vi "iLoveLangmuirProbes.vi"() -> ()   [LabVIEW 2022 SP3]
panel:
  out "Numeric":dbl
  out "Waveform Graph":dynamicdata(graph)
  out "XY Graph":cluster{"Y":dbl[], "Y":dbl[]}[](graph)
  out "VBias":dbl(knob) scale=-10.0..10.0
  in  "stop":bool
  out "VR":dbl(knob) scale=-10.0..10.0
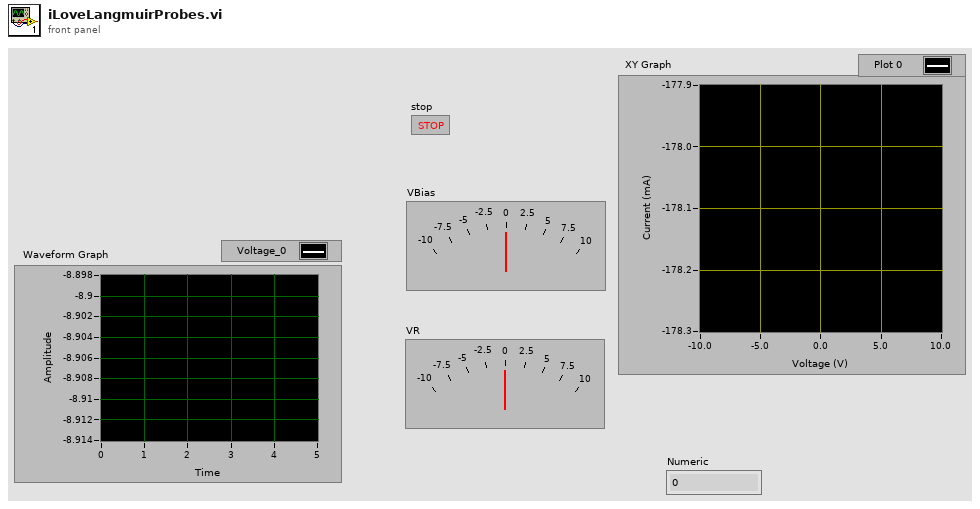
[diagram p1: front panel]
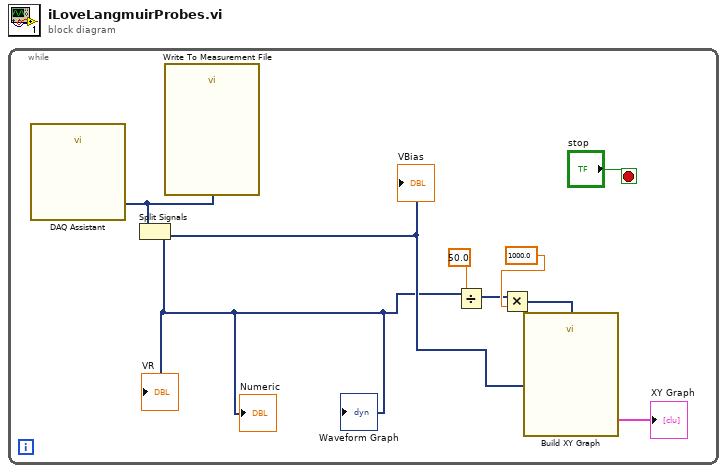
[diagram p0: block diagram]
diagram:
  n1 = while {
    stop <- "stop" stop-if-true
    n2 = call "DAQ Assistant"() -> ("data"=w3:dynamicdata)  [unwired: 17 in, 2 out]
    n3 = Split Signals(w3) -> (w1:dynamicdata, w2:dynamicdata)  [unwired: 2 in]
    "VR" <- w1
    "VBias" <- w2
    "Waveform Graph" <- w1
    "Numeric" <- w1
    n4 = call "Write To Measurement File"("Signals"=w3) -> ()  [unwired: 16 in, 3 out]
    n5 = Divide(x=w1, y=50.0) -> (x/y=w6:dynamicdata)
    n6 = Multiply(x=w6, y=1000.0) -> (x*y=w4:dynamicdata)
    n7 = call "Build XY Graph"("Y Input"=w4, "X Input"=w2) -> ("XY Graph"=→"XY Graph":cluster{"X":dbl[], "Y":dbl[]}[])  [unwired: 8 in, 1 out]
  }
